vi "Handle.vi"(7 "Event in":refnum<class "Event.lvclass">, 11 "Nominal State in":refnum<class "Nominal State.lvclass">) -> (2 "Destroy?":bool, 5 "Event out":refnum<class "Event.lvclass">)   [LabVIEW 2021, in "jettl.lvlib" / "Base Event.lvlib" / "State.lvlib" / "Nominal State.lvclass"]
uses:
  Nominal State.lvclass
  Event/Event.lvclass
  Nominal State.lvclass/Nominal State.ctl
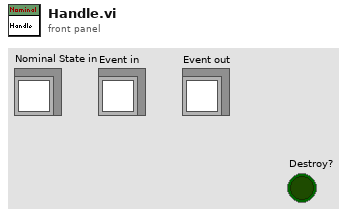
[diagram p1: front panel]
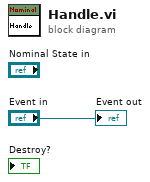
[diagram p0: block diagram]
diagram:
  "Event out" <- "Event in"
